vi "Update Number of Steps.vi"(10 "New Number of Steps":i32, 11 "UI Data in":refnum<class "Settings UI.lvclass">) -> (3 "UI Data in":refnum<class "Settings UI.lvclass">)   [LabVIEW 2024, in "Output Sequencer.lvlib" / "Settings UI.lvclass"]
uses:
  Settings UI.lvclass
  Settings UI.lvclass/Settings UI.ctl
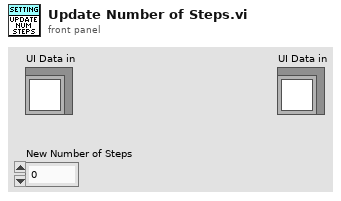
[diagram p1: front panel]
types:
  T1 = typedef "Output Sequencer.lvlib/Settings UI.lvclass/Step Settings.ctl" = cluster{"Description":string, "Precondition":string, "Duration":dbl, "Mode":string, "Delay Between Values":dbl, "Analog Values":string[], "Digital Values":string[], "Postcondition":string, "On True":string, "On False":string}
  T2 = map{i32, cluster{"Step Number":i32, "Description":string}}
  T3 = cluster{"Left Cell String":string, "Child Text":string[], "Child Tag":string, "Item Indent":i32, "Child Only?":bool, "Glyph Index":i32}[]
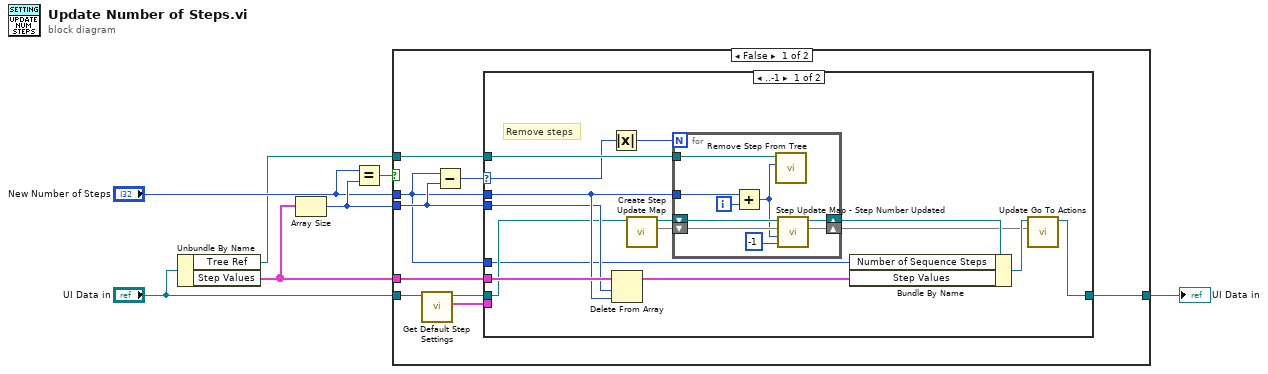
[diagram p0: block diagram]
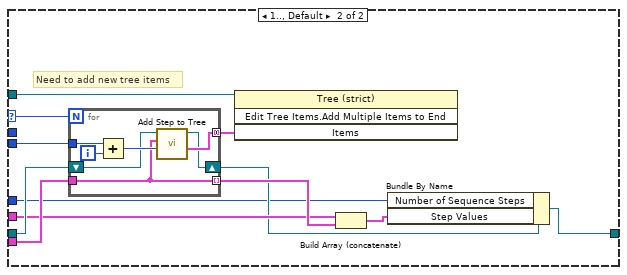
[diagram p2: hidden frame]
diagram:
  n1 = Unbundle By Name("UI Data in") -> ("Tree Ref"=w1:refnum<vi>, "Step Values"=w3:T1[])
  n2 = Array Size(array=w3) -> (size(s)=w5:i32)
  n3 = Equal?(x="New Number of Steps", y=w5) -> (x = y?=w2:bool)
  n4 = case shown="False" w2 {
    tunnel: w1 -> [w15 _]
    tunnel: w3 -> [w14 _]
    tunnel: "New Number of Steps" -> [w9 _]
    tunnel: w5 -> [w10 _]
    tunnel: "UI Data in" -> [w12 w60]
    tunnel: [w8 w60] -> w6
    frame False {
      n5 = call "Get Default Step Settings.vi"("UI Data In"=w12) -> ("Default Step Settings"=w13:T1, "UI Data out"=w11:refnum<class "Settings UI.lvclass">)  [unwired: 9 in]
      n6 = Subtract(x=w9, y=w10) -> (x-y=w16:i32)
      n7 = case shown="..-1" w16 {
        selector: w16 -> [w29 w46]
        tunnel: w15 -> [w30 w50]
        tunnel: w14 -> [w31 w47]
        tunnel: w9 -> [w28 _]
        tunnel: w10 -> [w26 w52]
        tunnel: w11 -> [w23 w51]
        tunnel: w13 -> [_ w49]
        tunnel: [w17 w41] -> w8
        tunnel: w9 -> [w21 w43]
        frame ..-1 {
          # "Remove steps"
          n8 = Absolute Value(x=w29) -> (abs(x)=w27:i32)
          n9 = Delete From Array(array=w31, length=w26, index=w28) -> (array with subset deleted=w20:T1[])  [unwired: 1 out]
          n10 = call "Create Step Update Map.vi"("Settings UI in"=w23) -> ("Step Update Map out"=w24:T2, "Settings UI out"=w25:refnum<class "Settings UI.lvclass">)  [unwired: 9 in]
          n11 = for {
            N: w27 -> [_]
            tunnel: w30 -> [w38]
            tunnel: w28 -> [w40]
            shift-right: [w33] -> w22
            shift-left: w25 -> [w36]
            shift-right: [w34] -> w18
            shift-left: w24 -> [w35]
            i -> [w39]
            n12 = Add(x=w40, y=w39) -> (x+y=w32:i32)
            n13 = call "Remove Step From Tree.vi"("Step Index"=w32, "TreeControl in"=w38) -> ()  [unwired: 9 in, 1 out]
            n14 = call "Step Update Map - Step Number Updated.vi"("New Step Number"=-1, "Previous Step Number"=w32, "Step Update Map in"=w35, "Settings UI in"=w36) -> ("Step Update Map out"=w34:T2, "Settings UI out"=w33:refnum<class "Settings UI.lvclass">)  [unwired: 6 in]
          }
          n15 = Bundle By Name(cluster=w22, "Number of Sequence Steps"=w21, "Step Values"=w20) -> (w19:refnum<class "Settings UI.lvclass">)
          n16 = call "Update Go To Actions.vi"("Step Update Map in"=w18, "Settings UI in"=w19) -> ("Settings UI out"=w17:refnum<class "Settings UI.lvclass">)  [unwired: 9 in]
        }
        frame 1.., Default {
          # "Need to add new tree items"
          n17 = for {
            N: w46 -> [_]
            tunnel: w52 -> [w59]
            tunnel: [w56] -> w45 mode=concatenating
            tunnel: w49 -> [w54]
            tunnel: [w54] -> w48 mode=indexing
            shift-right: [w53] -> w44
            shift-left: w51 -> [w55]
            i -> [w58]
            n18 = Add(x=w59, y=w58) -> (x+y=w57:i32)
            n19 = call "Add Step to Tree.vi"("Step Index"=w57, "Step Settings"=w54, "UI Data In"=w55) -> ("Tree Items"=w56:T3, "UI Data out"=w53:refnum<class "Settings UI.lvclass">)  [unwired: 6 in, 1 out]
          }
          n20 = invoke class="Tree (strict)" method="Edit Tree Items.Add Multiple Items to End"(reference=w50, "Items"=w45) -> ()  [unwired: 2 in, 4 out]
          n21 = Build Array (concatenate)(w47, w48) -> (w42:T1[])
          n22 = Bundle By Name(cluster=w44, "Number of Sequence Steps"=w43, "Step Values"=w42) -> (w41:refnum<class "Settings UI.lvclass">)
        }
      }
    }
    frame True {
    }
  }
  "UI Data in" <- w6
